vi "题目5.vi"() -> ()   [LabVIEW 2017]
panel:
  out "恭喜":bool
  out "通过":bool
  out "警告":bool
  in  "数值":i32
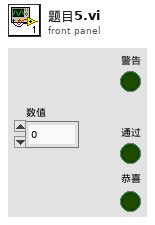
[diagram p1: front panel]
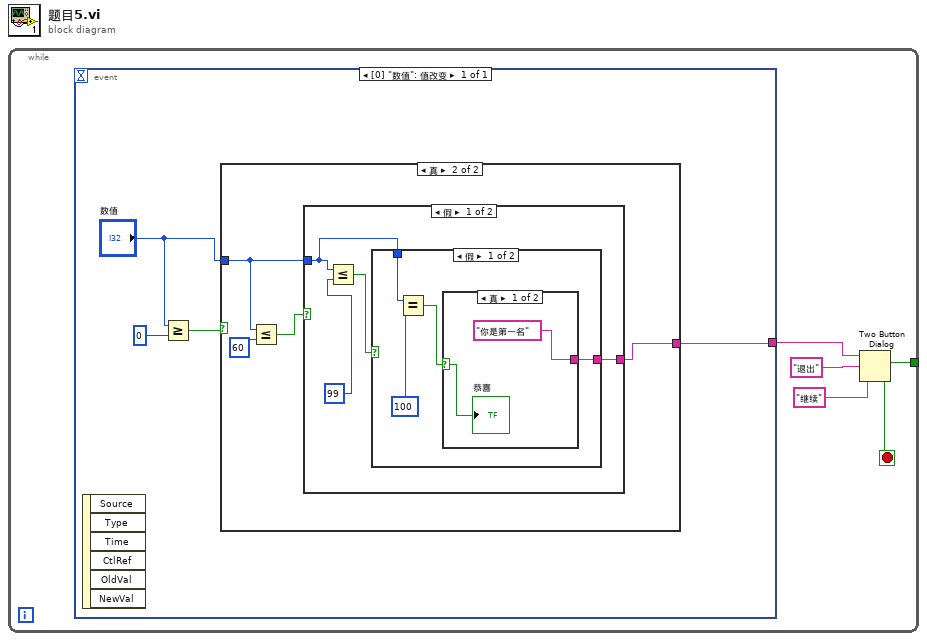
[diagram p0: block diagram]
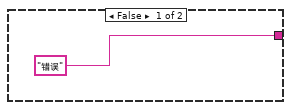
[diagram p2: hidden frame]
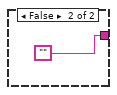
[diagram p3: hidden frame]
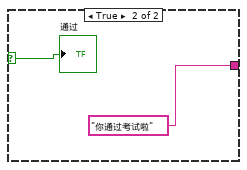
[diagram p4: hidden frame]
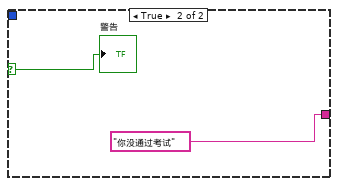
[diagram p5: hidden frame]
diagram:
  n1 = while {
    tunnel: [w2] -> _
    stop <- w2 stop-if-true
    n2 = event shown="[0] \"数值\": 值改变" {
      selector: _ -> [_]
      dyn-events: _ -> [_]
      timeout: _ -> [_]
      tunnel: [w6] -> w3
      event "数值": Value Change {
        n3 = event-data() -> ()  [unwired: 1 in, 6 out]
        n4 = Greater Or Equal?(x="数值", y=0) -> (x >= y?=w8:bool)
        n5 = case shown="真" w8 {
          tunnel: "数值" -> [_ w11]
          tunnel: ["错误" w10] -> w6
          frame False {
          }
          frame True {
            n6 = Less Or Equal?(x=w11, y=60) -> (x <= y?=w13:bool)
            n7 = case shown="假" w13 {
              selector: w13 -> [_ w28]
              tunnel: w11 -> [w15 _]
              tunnel: [w14 "你没通过考试"] -> w10
              frame False {
                n8 = Less Or Equal?(x=w15, y=99) -> (x <= y?=w16:bool)
                n9 = case shown="假" w16 {
                  selector: w16 -> [_ w26]
                  tunnel: w15 -> [w20 _]
                  tunnel: [w18 "你通过考试啦"] -> w14
                  frame False {
                    n10 = Equal?(x=w20, y=100) -> (x = y?=w19:bool)
                    n11 = case shown="真" w19 {
                      selector: w19 -> [w22 _]
                      tunnel: ["你是第一名" ""] -> w18
                      frame True {
                        "恭喜" <- w22
                      }
                      frame False {
                      }
                    }
                  }
                  frame True {
                    "通过" <- w26
                  }
                }
              }
              frame True {
                "警告" <- w28
              }
            }
          }
        }
      }
    }
    n12 = Two Button Dialog(message=w3, 1:"继续", 2:"退出") -> (T button?=w2:bool)
  }
